vi "Create Auto Config.vi"   [LabVIEW 2017]
uses:
  Routines and Block Data.ctl
  2018_Trobots_5013_Robot/Support Code/Blocks.ctl
types:
  T1 = typedef "Routines and Block Data.ctl" = cluster{"Routines":T2[][], "Block Data Array":variant[]}
  T2 = typedef "Blocks.ctl" = enum16{"", "Wait 1s", "Far--L", "L--end Sw", "end Sw--sq C1", "end cube --C1", "C1--d Hi", "C1--C3", "C3--C4", "d Hi--C1", "C3--end Sw", "C3--cube Sw", "M--front LSw", "M--front RSw", "front Sw--L", "L--C1", "C1--end cube"}
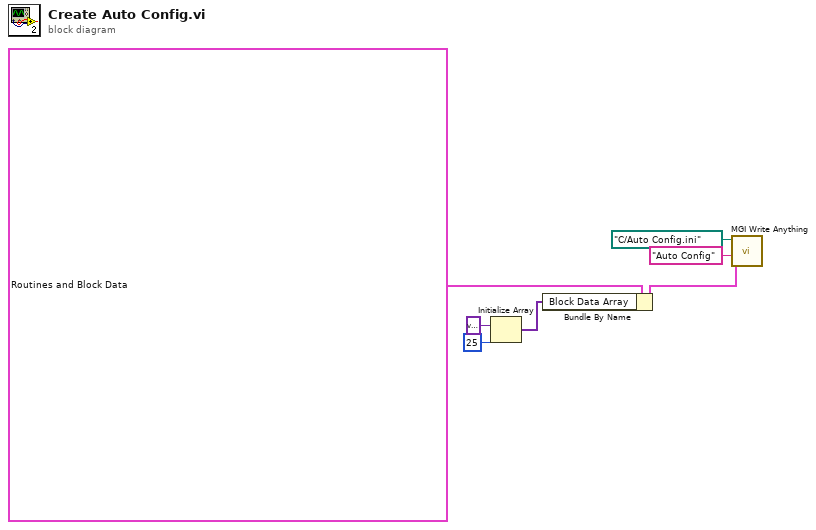
[diagram p0: block diagram]
diagram:
  n1 = Initialize Array(variant ("Block Data"), 25 ("dimension size")) -> (w1:variant[])
  n2 = Bundle By Name(cluster=T1 {"Routines"=array27x22[594 elements], "Block Data Array"=[]} ("Routines and Block Data"), "Block Data Array"=w1) -> (w4:T1)
  n3 = call <userlib>:"MGI Write Anything.vi"("Section Name (Name of \"Anything\")"="Auto Config" ("Section Name (Name of \"Anything\")"), "Anything"=w4, "Path (dialog)"=path "C:/Auto Config.ini") -> ()  [unwired: 6 in, 3 out]
